vi "Configure Acquisition.vi"(0 "VISA resource name":refnum<visa-resource-name>, 5 "Acquisition Type (0:Sample)":u16(ring) items=["Sample", "Peak Detect", "Hi Res", "Average", "Envelope", "WfmDB"], 7 "Average Waveforms (10)":i32=10, 9 "Envelope Waveforms (10)":i32=10, 11 "error in (no error)":errorcluster, 12 "WfmDB Samples (16000)":i32=16000, 13 "Sampling Modes (Real Time)":u16(ring) items=["Real Time", "Interpolater", "Equivalent"]) -> (4 "VISA resource name out":refnum<visa-resource-name>, 15 "error out":errorcluster)   [LabVIEW 2011, in "Tektronix 7000 Series.lvlib"]
doc: "Configures the acquisition method for an oscilloscope."
uses:
  Tektronix 7000 Series.lvlib
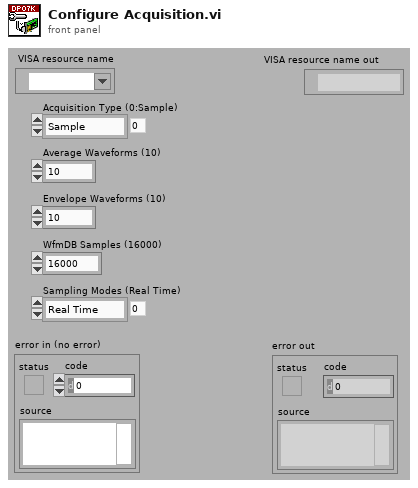
[diagram p1: front panel]
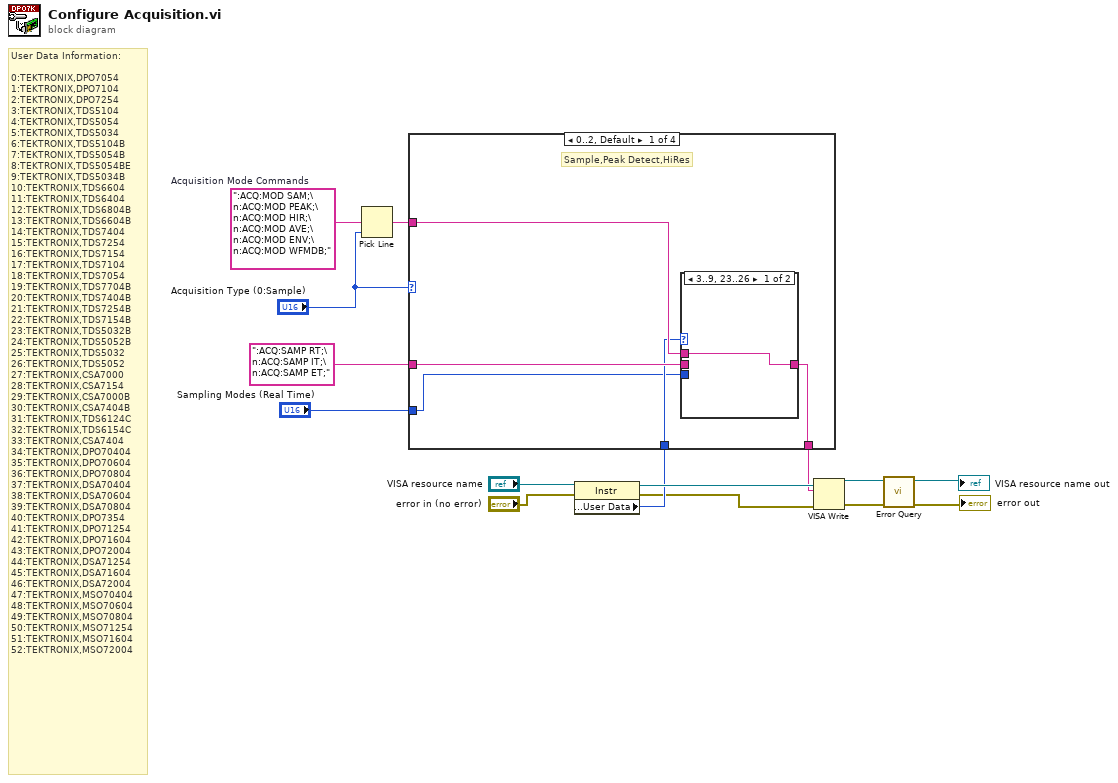
[diagram p0: block diagram]
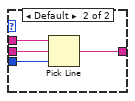
[diagram p2: hidden frame]
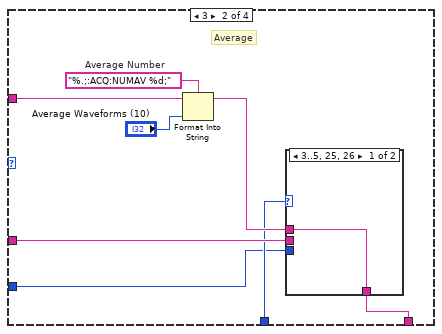
[diagram p3: hidden frame]
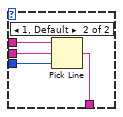
[diagram p4: hidden frame]
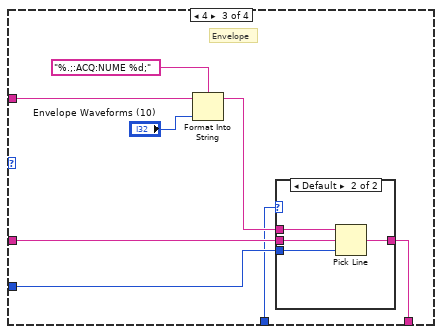
[diagram p5: hidden frame]
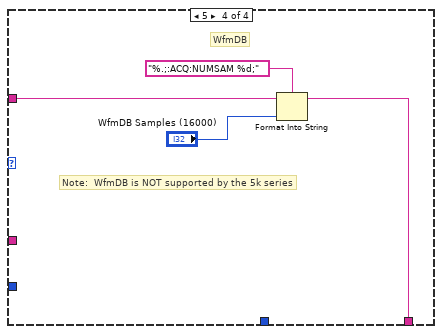
[diagram p7: hidden frame]
diagram:
  w15 = ":ACQ:MOD SAM;\n:ACQ:MOD PEAK;\n:ACQ:MOD HIR;\n:ACQ:MOD AVE;\n:ACQ:MOD ENV;\n:ACQ:MOD WFMDB;"  # Acquisition Mode Commands
  # "User Data Information:\n\n0:TEKTRONIX,DPO7054\n1:TEKTRONIX,DPO7104\n2:TEKTRONIX,DPO7254\n3:TEKTRONIX,TDS5104\n4:TEKTRONIX,TDS5054\n5:TEKTRONIX,TDS5034\n6:TEKTRONIX,TDS5104B\n7:TEKTRONIX,TDS5054B\n8:TEKTRONIX,TDS5054BE\n9:TEKTRONIX,TDS5034B\n10:TEKTRONIX,TDS6604\n11:TEKTRONIX,TDS6404\n12:TEKTRONIX,TDS6804B\n13:TEKTRONIX,TDS6604B\n14:TEKTRONIX,TDS7404\n15:TEKTRONIX,TDS7254\n16:TEKTRONIX,TDS7154\n17:TEKTRONIX,TDS7104\n18:TEKTRONIX,TDS7054\n19:TEKTRONIX,TDS7704B\n20:TEKTRONIX,TDS7404B\n21:TEKTRONIX,TDS7254B\n22:TEKTRONIX,TDS7154B\n23:TEKTRONIX,TDS5032B\n24:TEKTRONIX,TDS5052B\n25:TEKTRONIX,TDS5032\n26:TEKTRONIX,TDS5052\n27:TEKTRONIX,CSA7000\n28:TEKTRONIX,CSA7154\n29:TEKTRONIX,CSA7000B\n30:TEKTRONIX,CSA7404B\n31:TEKTRONIX,TDS6124C\n32:TEKTRONIX,TDS6154C\n33:TEKTRONIX,CSA7404\n34:TEKTRONIX,DPO70404\n35:TEKTRONIX,DPO70604\n36:TEKTRONIX,DPO70804\n37:TEKTRONIX,DSA70404\n38:TEKTRONIX,DSA70604\n39:TEKTRONIX,DSA70804\n40:TEKTRONIX,DPO7354\n41:TEKTRONIX,DPO71254\n42:TEKTRONIX,DPO71604\n43:TEKTRONIX,DPO72004\n44:TEKTRONIX,DSA71254\n45:TEKTRONIX,DSA71604\n46:TEKTRONIX,DSA72004\n47:TEKTRONIX,MSO70404\n48:TEKTRONIX,MSO70604\n49:TEKTRONIX,MSO70804\n50:TEKTRONIX,MSO71254\n51:TEKTRONIX,MSO71604\n52:TEKTRONIX,MSO72004"
  n1 = Pick Line(multi-line string=w15, line index="Acquisition Type (0:Sample)") -> (output string=w14:string)  [unwired: 1 in]
  n2 = property class="Instr"(reference="VISA resource name", error in="error in (no error)") -> (reference out=w5:refnum<visa-resource-name>, error out=w3:errorcluster, "General Settings:User Data"=w4:u32)
  n3 = case shown="0..2, Default" "Acquisition Type (0:Sample)" {
    tunnel: w14 -> [w20 w33 w46 w55]
    tunnel: ":ACQ:SAMP RT;\n:ACQ:SAMP IT;\n:ACQ:SAMP ET;" -> [w19 w29 w43 _]
    tunnel: [w18 w26 w41 w52] -> w2
    tunnel: w4 -> [w17 w28 w39 _]
    tunnel: "Sampling Modes (Real Time)" -> [w16 w27 w40 _]
    frame 0..2, Default {
      # "Sample,Peak Detect,HiRes"
      n4 = case shown="3..9, 23..26" w17 {
        tunnel: w20 -> [w21 w22]
        tunnel: w19 -> [_ w25]
        tunnel: w16 -> [_ w24]
        tunnel: [w21 w23] -> w18
        frame 3..9, 23..26 {
        }
        frame Default {
          n5 = Pick Line(string ("")=w22, multi-line string=w25, line index=w24) -> (output string=w23:string)
        }
      }
    }
    frame 3 {
      w32 = "%.;:ACQ:NUMAV %d;"  # Average Number
      # "Average"
      n6 = Format Into String(format string=w32, initial string=w33, "Average Waveforms (10)") -> (resulting string=w30:string)  [unwired: 1 in, 1 out]
      n7 = case shown="3..5, 25, 26" w28 {
        tunnel: w30 -> [w34 w38]
        tunnel: w29 -> [_ w37]
        tunnel: w27 -> [_ w36]
        tunnel: [w34 w35] -> w26
        frame 3..5, 25, 26 {
        }
        frame 1, Default {
          n8 = Pick Line(string ("")=w38, multi-line string=w37, line index=w36) -> (output string=w35:string)
        }
      }
    }
    frame 4 {
      # "Envelope"
      n9 = Format Into String(format string="%.;:ACQ:NUME %d;", initial string=w46, "Envelope Waveforms (10)") -> (resulting string=w42:string)  [unwired: 1 in, 1 out]
      n10 = case shown="Default" w39 {
        tunnel: w43 -> [_ w51]
        tunnel: w42 -> [w47 w50]
        tunnel: [w47 w49] -> w41
        tunnel: w40 -> [_ w48]
        frame 3..9, 23..26 {
        }
        frame Default {
          n11 = Pick Line(string ("")=w50, multi-line string=w51, line index=w48) -> (output string=w49:string)
        }
      }
    }
    frame 5 {
      # "Note:  WfmDB is NOT supported by the 5k series"
      # "WfmDB"
      n12 = Format Into String(format string="%.;:ACQ:NUMSAM %d;", initial string=w55, "WfmDB Samples (16000)") -> (resulting string=w52:string)  [unwired: 1 in, 1 out]
    }
  }
  n13 = VISA Write(VISA resource name=w5, write buffer=w2, error in (no error)=w3) -> (VISA resource name out=w13:refnum<visa-resource-name>, error out=w11:errorcluster)  [unwired: 1 out]
  n14 = call "Error Query.vi"("error in (no error)"=w11, "VISA resource name"=w13) -> ("error out"=→"error out":errorcluster, "VISA resource name out"=→"VISA resource name out":refnum<visa-resource-name>)  [unwired: 6 in, 2 out]
